vi "Read Assert Data.vi"(11 "Message Assertion":refnum<class "TestManagerMsg.Assertion.lvclass">) -> (2 "Assert Data":T1={"Label"="", "Asserted"=FALSE, "call-chain"=[], "upstream-error"={"status"=FALSE, "code"=0, "source"=""}, "timestamp"=timestamp(0 s since 1904-01-01), "Execution time (s)"=-1.0}, 3 "Message Assertion out":refnum<class "TestManagerMsg.Assertion.lvclass">)   [LabVIEW 2013, in "Caraya.lvlib" / "TestManagerMsg.Assertion.lvclass"]
uses:
  TestManagerMsg.Assertion.lvclass
  Assert-Data -- cluster.ctl
  TestManagerMsg.Assertion.lvclass/TestManagerMsg.Assertion.ctl
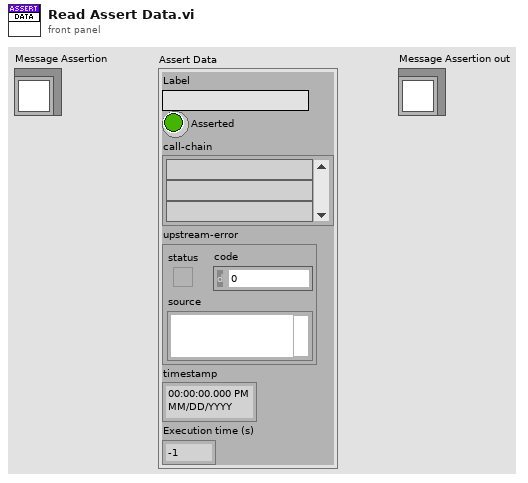
[diagram p1: front panel]
types:
  T1 = typedef "Caraya.lvlib/TestManagerMsg.Assertion.lvclass/Assert-Data -- cluster.ctl" = cluster{"Label":string, "Asserted":bool, "call-chain":string[], "upstream-error":errorcluster, "timestamp":timestamp, "Execution time (s)":dbl}
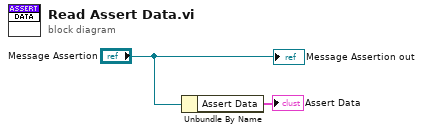
[diagram p0: block diagram]
diagram:
  n1 = Unbundle By Name("Message Assertion") -> ("Assert Data"=→"Assert Data":T1)
  "Message Assertion out" <- "Message Assertion"
